vi "processMenuSelection.vi"(8 "eventData":T1, 10 "ItemPath":string, 11 "queues":T2) -> (0 "eventData 2":T1)   [LabVIEW 2018]
uses:
  Queues.ctl
  event data.ctl
  <vilib>/LabVIEW Targets/FPGA/cRIO/shared/nicrio_ModuleControls/nicrio_cRIO-9237_DataRatesRing.ctl
  supporting VIs/polymorphic VIs/enqueue for message handler.vi
  supporting VIs/polymorphic VIs/enqueue for user interface.vi
  supporting VIs/polymorphic VIs/enqueue for data processor.vi
  supporting VIs/polymorphic VIs/enqueue for file IO.vi
  RT/Message Handler loop/FPGA commands/RT - FPGA commands.lvlib
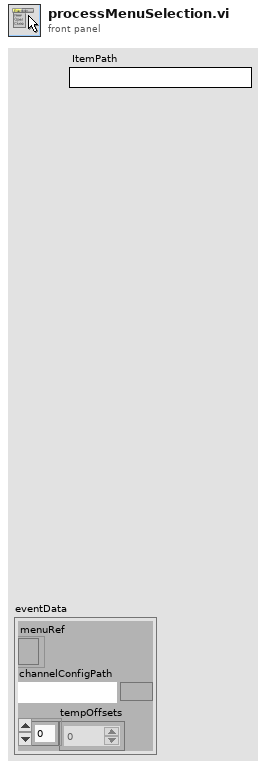
[diagram p1: front panel]
types:
  T1 = typedef "event data.ctl" = cluster{"menuRef":refnum<k9>, "channelConfigPath":path, "tempOffsets":dbl[]}
  T2 = typedef "Queues.ctl" = cluster{"messageHandler":refnum<queue>, "comms":refnum<queue>, "dataStream":refnum<queue>, "dataProcessor":refnum<queue>, "fileIO":refnum<queue>, "userInterface":refnum<queue>, "errors":refnum<queue>, "customCompressor":refnum<queue>}
  T3 = typedef "nicrio_cRIO-9237_DataRatesRing.ctl" = u8
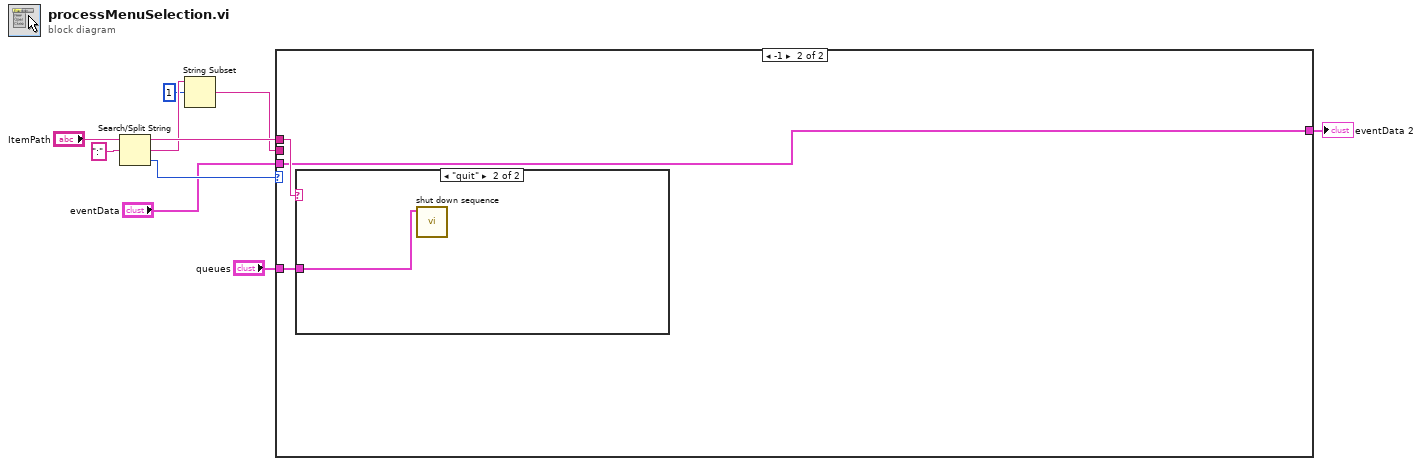
[diagram p0: block diagram]
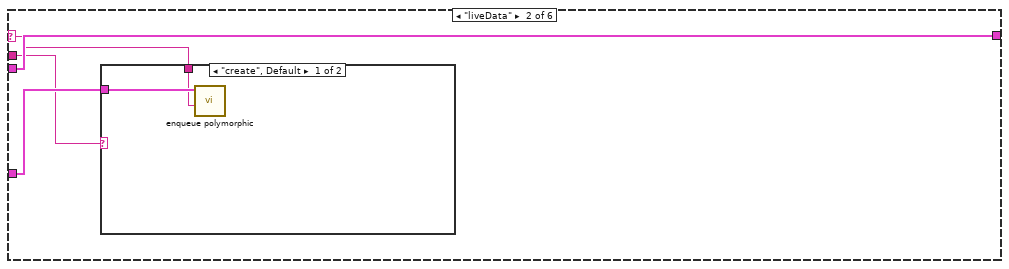
[diagram p3: hidden frame]
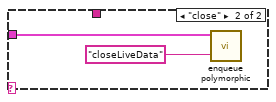
[diagram p4: hidden frame]
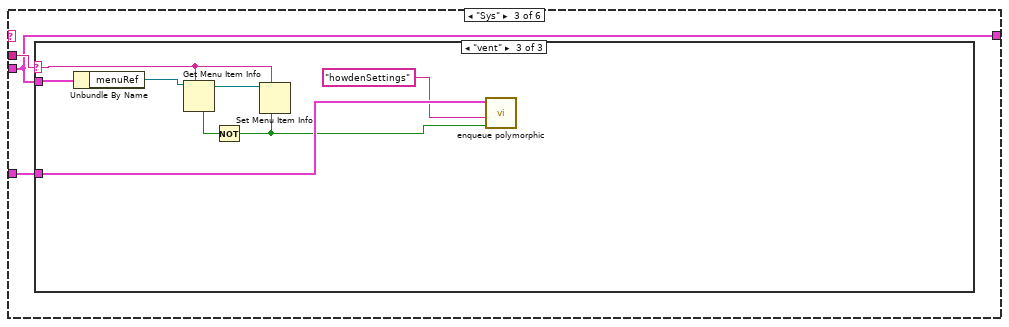
[diagram p5: hidden frame]
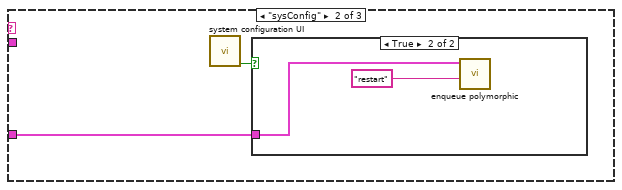
[diagram p7: hidden frame]
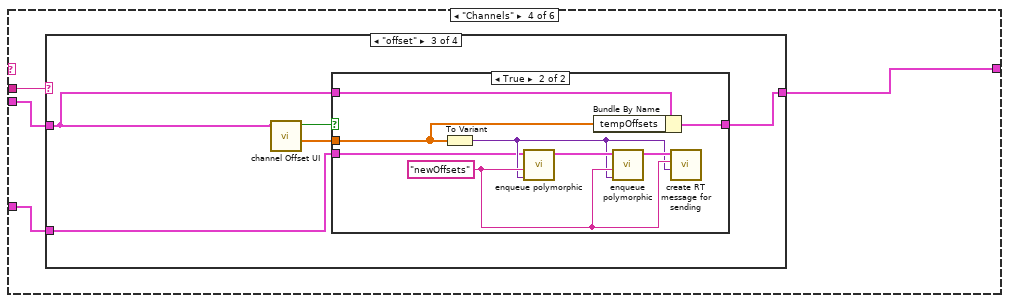
[diagram p9: hidden frame]
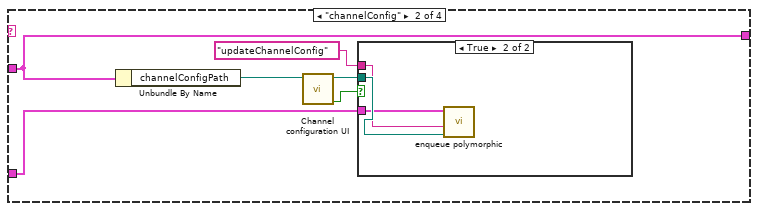
[diagram p11: hidden frame]
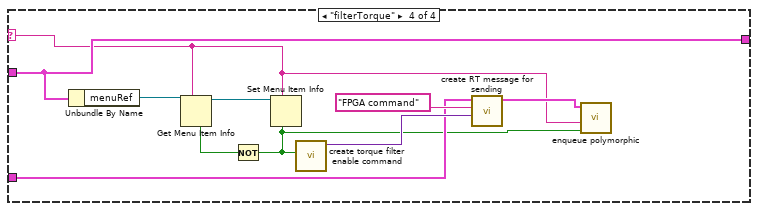
[diagram p14: hidden frame]
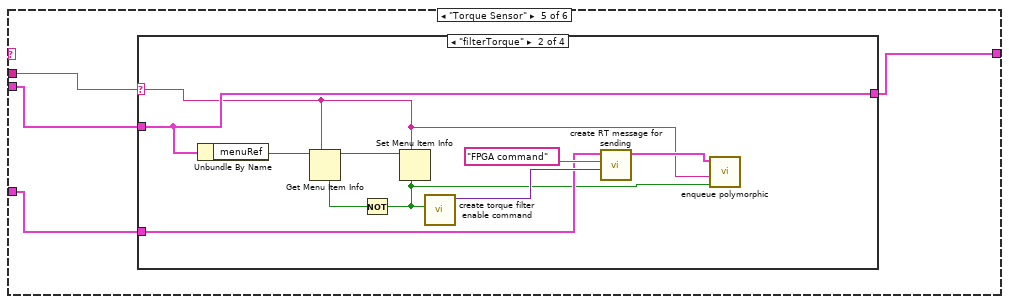
[diagram p15: hidden frame]
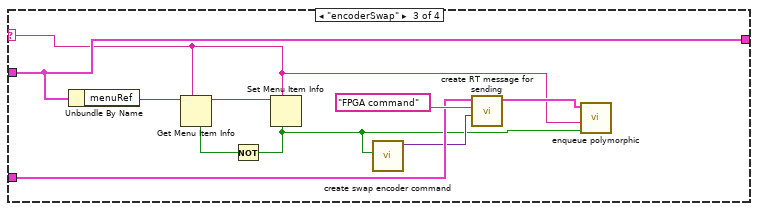
[diagram p17: hidden frame]
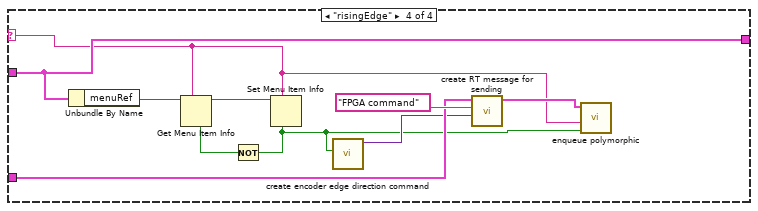
[diagram p18: hidden frame]
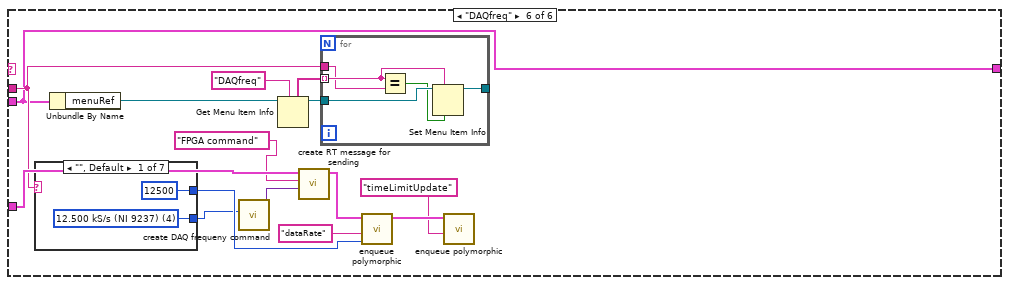
[diagram p19: hidden frame]
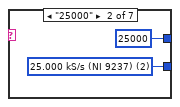
[diagram p20: hidden frame]
diagram:
  n1 = Search/Split String(string="ItemPath", search string/char (-)=":") -> (substring before match=w6:string, match + rest of string=w5:string, offset of match=w7:i32)  [unwired: 1 in]
  n2 = String Subset(string=w5, offset (0)=1) -> (substring=w3:string)  [unwired: 1 in]
  n3 = case shown="-1" w7 {
    tunnel: "queues" -> [w13 w149]
    tunnel: "eventData" -> [w12 w147]
    tunnel: w6 -> [w15 w148]
    tunnel: w3 -> [w14 _]
    tunnel: [w11 w147] -> w1
    frame 0, Default {
      n4 = case shown="\"\", Default" w15 {
        selector: w15 -> [_ w18 _ _ _ _]
        tunnel: w14 -> [_ w17 w26 w42 w79 w122]
        tunnel: w13 -> [_ w19 w27 w43 w81 w127]
        tunnel: w12 -> [w16 w20 w25 w41 w80 w121]
        tunnel: [w16 w20 w25 w40 w78 w121] -> w11
        frame "", Default {
        }
        frame "liveData" {
          n5 = case shown="\"create\", Default" w17 {
            tunnel: w19 -> [w22 w24]
            tunnel: w18 -> [w21 _]
            frame "create", Default {
              n6 = call-poly "enqueue polymorphic.vi"("message"=w21, "Queues"=w22) -> ()  [unwired: 9 in, 1 out]
            }
            frame "close" {
              n7 = call-poly "enqueue polymorphic.vi"("message"="closeLiveData", "Queues"=w24) -> ()  [unwired: 9 in, 1 out]
            }
          }
        }
        frame "Sys" {
          n8 = case shown="\"vent\"" w26 {
            selector: w26 -> [_ _ w34]
            tunnel: w27 -> [_ w28 w39]
            tunnel: w25 -> [_ _ w38]
            frame "", Default {
            }
            frame "sysConfig" {
              n9 = call "system configuration UI.vi"() -> ("file updated"=w29:bool)  [unwired: 11 in]
              n10 = case shown="True" w29 {
                tunnel: w28 -> [_ w30]
                frame False {
                }
                frame True {
                  n11 = call-poly "enqueue polymorphic.vi"("message"="restart" ("F button name (\"Cancel\")"), "Queues"=w30) -> ()  [unwired: 9 in, 1 out]
                }
              }
            }
            frame "vent" {
              n12 = Unbundle By Name(w38) -> ("menuRef"=w37:refnum<k9>)
              n13 = Get Menu Item Info(7:w34, 11:w37) -> (3:w32:refnum<k9>, 4:w35:bool)  [unwired: 1 in, 5 out]
              n14 = Not(x=w35) -> (.not. x?=w33:bool)
              n15 = Set Menu Item Info(6:w33, 7:w34, 11:w32) -> ()  [unwired: 4 in, 2 out]
              n16 = call-poly "enqueue polymorphic.vi"("data"=w33, "message"="howdenSettings" ("F button name (\"Cancel\")"), "Queues"=w39) -> ()  [unwired: 8 in, 1 out]
            }
          }
        }
        frame "Channels" {
          n17 = case shown="\"offset\"" w42 {
            selector: w42 -> [_ _ _ w70]
            tunnel: w43 -> [_ w46 w57 w72]
            tunnel: w41 -> [w44 w45 w54 w77]
            tunnel: [w44 w45 w55 w77] -> w40
            frame "", Default {
            }
            frame "channelConfig" {
              n18 = Unbundle By Name(w45) -> ("channelConfigPath"=w47:path)
              n19 = call "Channel configuration UI.vi"("config file"=w47) -> ("updated?"=w48:bool, "Current config file:"=w50:path)  [unwired: 9 in]
              n20 = case shown="True" w48 {
                tunnel: w50 -> [_ w53]
                tunnel: w46 -> [_ w52]
                tunnel: "updateChannelConfig" ("message") -> [_ w51]
                frame False {
                }
                frame True {
                  n21 = call-poly "enqueue polymorphic.vi"("data"=w53, "message"=w51, "Queues"=w52) -> ()  [unwired: 8 in, 1 out]
                }
              }
            }
            frame "offset" {
              n22 = call "channel Offset UI.vi"("eventData"=w54) -> ("offsets"=w56:dbl[], "changed?"=w58:bool)  [unwired: 9 in]
              n23 = case shown="True" w58 {
                tunnel: w56 -> [_ w60]
                tunnel: w57 -> [_ w63]
                tunnel: w54 -> [w59 w62]
                tunnel: [w59 w61] -> w55
                frame False {
                }
                frame True {
                  w65 = "newOffsets" ("message")
                  n24 = To Variant(anything=w60) -> (Variant=w64:variant)
                  n25 = call-poly "enqueue polymorphic.vi"("data"=w64, "message"=w65, "Queues"=w63) -> ("Queues out"=w67:T2)  [unwired: 8 in]
                  n26 = Bundle By Name(cluster=w62, "tempOffsets"=w60) -> (w61:T1)
                  n27 = call-poly "enqueue polymorphic.vi"("data"=w64, "message"=w65, "Queues"=w67) -> ("Queues out"=w66:T2)  [unwired: 8 in]
                  n28 = call "create RT message for sending.vi"("RT data"=w64, "RT message"=w65, "Queues in"=w66) -> ()  [unwired: 8 in, 1 out]
                }
              }
            }
            frame "filterTorque" {
              n29 = Unbundle By Name(w77) -> ("menuRef"=w68:refnum<k9>)
              n30 = Get Menu Item Info(7:w70, 11:w68) -> (3:w75:refnum<k9>, 4:w76:bool)  [unwired: 1 in, 5 out]
              n31 = Not(x=w76) -> (.not. x?=w69:bool)
              n32 = Set Menu Item Info(6:w69, 7:w70, 11:w75) -> ()  [unwired: 4 in, 2 out]
              n33 = call "create torque filter enable command.vi"("Enable filter"=w69) -> ("command message"=w74:variant)  [unwired: 10 in]
              n34 = call "create RT message for sending.vi"("RT data"=w74, "RT message"="FPGA command", "Queues in"=w72) -> ("Queues out"=w71:T2)  [unwired: 8 in]
              n35 = call-poly "enqueue polymorphic.vi"("data"=w69, "message"=w70, "Queues"=w71) -> ()  [unwired: 8 in, 1 out]
            }
          }
        }
        frame "Torque Sensor" {
          n36 = case shown="\"filterTorque\"" w79 {
            selector: w79 -> [_ w84 w95 w105]
            tunnel: w81 -> [_ w86 w97 w107]
            tunnel: w80 -> [w82 w92 w102 w112]
            tunnel: [w82 w92 w102 w112] -> w78
            frame "", Default {
            }
            frame "filterTorque" {
              n37 = Unbundle By Name(w92) -> ("menuRef"=w91:refnum<k9>)
              n38 = Get Menu Item Info(7:w84, 11:w91) -> (3:w89:refnum<k9>, 4:w90:bool)  [unwired: 1 in, 5 out]
              n39 = Not(x=w90) -> (.not. x?=w83:bool)
              n40 = Set Menu Item Info(6:w83, 7:w84, 11:w89) -> ()  [unwired: 4 in, 2 out]
              n41 = call "create torque filter enable command.vi"("Enable filter"=w83) -> ("command message"=w88:variant)  [unwired: 10 in]
              n42 = call "create RT message for sending.vi"("RT data"=w88, "RT message"="FPGA command", "Queues in"=w86) -> ("Queues out"=w85:T2)  [unwired: 8 in]
              n43 = call-poly "enqueue polymorphic.vi"("data"=w83, "message"=w84, "Queues"=w85) -> ()  [unwired: 8 in, 1 out]
            }
            frame "encoderSwap" {
              n44 = Unbundle By Name(w102) -> ("menuRef"=w101:refnum<k9>)
              n45 = Get Menu Item Info(7:w95, 11:w101) -> (3:w99:refnum<k9>, 4:w100:bool)  [unwired: 1 in, 5 out]
              n46 = Not(x=w100) -> (.not. x?=w93:bool)
              n47 = Set Menu Item Info(6:w93, 7:w95, 11:w99) -> ()  [unwired: 4 in, 2 out]
              n48 = call "create swap encoder command.vi"("swap encoders"=w93) -> ("command message"=w94:variant)  [unwired: 10 in]
              n49 = call "create RT message for sending.vi"("RT data"=w94, "RT message"="FPGA command", "Queues in"=w97) -> ("Queues out"=w96:T2)  [unwired: 8 in]
              n50 = call-poly "enqueue polymorphic.vi"("data"=w93, "message"=w95, "Queues"=w96) -> ()  [unwired: 8 in, 1 out]
            }
            frame "risingEdge" {
              n51 = Unbundle By Name(w112) -> ("menuRef"=w111:refnum<k9>)
              n52 = Get Menu Item Info(7:w105, 11:w111) -> (3:w109:refnum<k9>, 4:w110:bool)  [unwired: 1 in, 5 out]
              n53 = Not(x=w110) -> (.not. x?=w103:bool)
              n54 = Set Menu Item Info(6:w103, 7:w105, 11:w109) -> ()  [unwired: 4 in, 2 out]
              n55 = call "create encoder edge direction command.vi"("Falling edge?"=w103) -> ("command message"=w104:variant)  [unwired: 10 in]
              n56 = call "create RT message for sending.vi"("RT data"=w104, "RT message"="FPGA command", "Queues in"=w107) -> ("Queues out"=w106:T2)  [unwired: 8 in]
              n57 = call-poly "enqueue polymorphic.vi"("data"=w103, "message"=w105, "Queues"=w106) -> ()  [unwired: 8 in, 1 out]
            }
          }
        }
        frame "DAQfreq" {
          n58 = case shown="\"\", Default" w122 {
            tunnel: [u16 12500 u16 25000 u16 12500 u16 10000 u16 5000 u16 2500 u16 2000] -> w120
            tunnel: [w134 w135 w137 w140 w141 w143 w145] -> w117
            frame "", Default {
              w134 = T3 4 items=["50.000 kS/s (NI 9237)"=1, "25.000 kS/s (NI 9237)"=2, "16.667 kS/s (NI 9237)"=3, "12.500 kS/s (NI 9237)"=4, "10.000 kS/s (NI 9237)"=5, "8.333 kS/s (NI 9237)"=6, "7.143 kS/s (NI 9237)"=7, "6.250 kS/s (NI 9237)"=8, "5.556 kS/s (NI 9237)"=9, "5.000 kS/s (NI 9237)"=10, "4.545 kS/s (NI 9237)"=11, "4.167 kS/s (NI 9237)"=12, "3.846 kS/s (NI 9237)"=13, "3.571 kS/s (NI 9237)"=14, "3.333 kS/s (NI 9237)"=15, "3.125 kS/s (NI 9237)"=16, "2.941 kS/s (NI 9237)"=17, "2.778 kS/s (NI 9237)"=18, "2.632 kS/s (NI 9237)"=19, "2.500 kS/s (NI 9237)"=20, "2.381 kS/s (NI 9237)"=21, "2.273 kS/s (NI 9237)"=22, "2.174 kS/s (NI 9237)"=23, "2.083 kS/s (NI 9237)"=24, "2.000 kS/s (NI 9237)"=25, "1.923 kS/s (NI 9237)"=26, "1.852 kS/s (NI 9237)"=27, "1.786 kS/s (NI 9237)"=28, "1.724 kS/s (NI 9237)"=29, "1.667 kS/s (NI 9237)"=30, "1.613 kS/s (NI 9237)"=31] ("Data Rate")
            }
            frame "25000" {
              w135 = T3 2 items=["50.000 kS/s (NI 9237)"=1, "25.000 kS/s (NI 9237)"=2, "16.667 kS/s (NI 9237)"=3, "12.500 kS/s (NI 9237)"=4, "10.000 kS/s (NI 9237)"=5, "8.333 kS/s (NI 9237)"=6, "7.143 kS/s (NI 9237)"=7, "6.250 kS/s (NI 9237)"=8, "5.556 kS/s (NI 9237)"=9, "5.000 kS/s (NI 9237)"=10, "4.545 kS/s (NI 9237)"=11, "4.167 kS/s (NI 9237)"=12, "3.846 kS/s (NI 9237)"=13, "3.571 kS/s (NI 9237)"=14, "3.333 kS/s (NI 9237)"=15, "3.125 kS/s (NI 9237)"=16, "2.941 kS/s (NI 9237)"=17, "2.778 kS/s (NI 9237)"=18, "2.632 kS/s (NI 9237)"=19, "2.500 kS/s (NI 9237)"=20, "2.381 kS/s (NI 9237)"=21, "2.273 kS/s (NI 9237)"=22, "2.174 kS/s (NI 9237)"=23, "2.083 kS/s (NI 9237)"=24, "2.000 kS/s (NI 9237)"=25, "1.923 kS/s (NI 9237)"=26, "1.852 kS/s (NI 9237)"=27, "1.786 kS/s (NI 9237)"=28, "1.724 kS/s (NI 9237)"=29, "1.667 kS/s (NI 9237)"=30, "1.613 kS/s (NI 9237)"=31] ("Data Rate")
            }
            frame "12500" {
              w137 = T3 4 items=["50.000 kS/s (NI 9237)"=1, "25.000 kS/s (NI 9237)"=2, "16.667 kS/s (NI 9237)"=3, "12.500 kS/s (NI 9237)"=4, "10.000 kS/s (NI 9237)"=5, "8.333 kS/s (NI 9237)"=6, "7.143 kS/s (NI 9237)"=7, "6.250 kS/s (NI 9237)"=8, "5.556 kS/s (NI 9237)"=9, "5.000 kS/s (NI 9237)"=10, "4.545 kS/s (NI 9237)"=11, "4.167 kS/s (NI 9237)"=12, "3.846 kS/s (NI 9237)"=13, "3.571 kS/s (NI 9237)"=14, "3.333 kS/s (NI 9237)"=15, "3.125 kS/s (NI 9237)"=16, "2.941 kS/s (NI 9237)"=17, "2.778 kS/s (NI 9237)"=18, "2.632 kS/s (NI 9237)"=19, "2.500 kS/s (NI 9237)"=20, "2.381 kS/s (NI 9237)"=21, "2.273 kS/s (NI 9237)"=22, "2.174 kS/s (NI 9237)"=23, "2.083 kS/s (NI 9237)"=24, "2.000 kS/s (NI 9237)"=25, "1.923 kS/s (NI 9237)"=26, "1.852 kS/s (NI 9237)"=27, "1.786 kS/s (NI 9237)"=28, "1.724 kS/s (NI 9237)"=29, "1.667 kS/s (NI 9237)"=30, "1.613 kS/s (NI 9237)"=31] ("Data Rate")
            }
            frame "10000" {
              w140 = T3 5 items=["50.000 kS/s (NI 9237)"=1, "25.000 kS/s (NI 9237)"=2, "16.667 kS/s (NI 9237)"=3, "12.500 kS/s (NI 9237)"=4, "10.000 kS/s (NI 9237)"=5, "8.333 kS/s (NI 9237)"=6, "7.143 kS/s (NI 9237)"=7, "6.250 kS/s (NI 9237)"=8, "5.556 kS/s (NI 9237)"=9, "5.000 kS/s (NI 9237)"=10, "4.545 kS/s (NI 9237)"=11, "4.167 kS/s (NI 9237)"=12, "3.846 kS/s (NI 9237)"=13, "3.571 kS/s (NI 9237)"=14, "3.333 kS/s (NI 9237)"=15, "3.125 kS/s (NI 9237)"=16, "2.941 kS/s (NI 9237)"=17, "2.778 kS/s (NI 9237)"=18, "2.632 kS/s (NI 9237)"=19, "2.500 kS/s (NI 9237)"=20, "2.381 kS/s (NI 9237)"=21, "2.273 kS/s (NI 9237)"=22, "2.174 kS/s (NI 9237)"=23, "2.083 kS/s (NI 9237)"=24, "2.000 kS/s (NI 9237)"=25, "1.923 kS/s (NI 9237)"=26, "1.852 kS/s (NI 9237)"=27, "1.786 kS/s (NI 9237)"=28, "1.724 kS/s (NI 9237)"=29, "1.667 kS/s (NI 9237)"=30, "1.613 kS/s (NI 9237)"=31] ("Data Rate")
            }
            frame "5000" {
              w141 = T3 10 items=["50.000 kS/s (NI 9237)"=1, "25.000 kS/s (NI 9237)"=2, "16.667 kS/s (NI 9237)"=3, "12.500 kS/s (NI 9237)"=4, "10.000 kS/s (NI 9237)"=5, "8.333 kS/s (NI 9237)"=6, "7.143 kS/s (NI 9237)"=7, "6.250 kS/s (NI 9237)"=8, "5.556 kS/s (NI 9237)"=9, "5.000 kS/s (NI 9237)"=10, "4.545 kS/s (NI 9237)"=11, "4.167 kS/s (NI 9237)"=12, "3.846 kS/s (NI 9237)"=13, "3.571 kS/s (NI 9237)"=14, "3.333 kS/s (NI 9237)"=15, "3.125 kS/s (NI 9237)"=16, "2.941 kS/s (NI 9237)"=17, "2.778 kS/s (NI 9237)"=18, "2.632 kS/s (NI 9237)"=19, "2.500 kS/s (NI 9237)"=20, "2.381 kS/s (NI 9237)"=21, "2.273 kS/s (NI 9237)"=22, "2.174 kS/s (NI 9237)"=23, "2.083 kS/s (NI 9237)"=24, "2.000 kS/s (NI 9237)"=25, "1.923 kS/s (NI 9237)"=26, "1.852 kS/s (NI 9237)"=27, "1.786 kS/s (NI 9237)"=28, "1.724 kS/s (NI 9237)"=29, "1.667 kS/s (NI 9237)"=30, "1.613 kS/s (NI 9237)"=31] ("Data Rate")
            }
            frame "2500" {
              w143 = T3 20 items=["50.000 kS/s (NI 9237)"=1, "25.000 kS/s (NI 9237)"=2, "16.667 kS/s (NI 9237)"=3, "12.500 kS/s (NI 9237)"=4, "10.000 kS/s (NI 9237)"=5, "8.333 kS/s (NI 9237)"=6, "7.143 kS/s (NI 9237)"=7, "6.250 kS/s (NI 9237)"=8, "5.556 kS/s (NI 9237)"=9, "5.000 kS/s (NI 9237)"=10, "4.545 kS/s (NI 9237)"=11, "4.167 kS/s (NI 9237)"=12, "3.846 kS/s (NI 9237)"=13, "3.571 kS/s (NI 9237)"=14, "3.333 kS/s (NI 9237)"=15, "3.125 kS/s (NI 9237)"=16, "2.941 kS/s (NI 9237)"=17, "2.778 kS/s (NI 9237)"=18, "2.632 kS/s (NI 9237)"=19, "2.500 kS/s (NI 9237)"=20, "2.381 kS/s (NI 9237)"=21, "2.273 kS/s (NI 9237)"=22, "2.174 kS/s (NI 9237)"=23, "2.083 kS/s (NI 9237)"=24, "2.000 kS/s (NI 9237)"=25, "1.923 kS/s (NI 9237)"=26, "1.852 kS/s (NI 9237)"=27, "1.786 kS/s (NI 9237)"=28, "1.724 kS/s (NI 9237)"=29, "1.667 kS/s (NI 9237)"=30, "1.613 kS/s (NI 9237)"=31] ("Data Rate")
            }
            frame "2000" {
              w145 = T3 25 items=["50.000 kS/s (NI 9237)"=1, "25.000 kS/s (NI 9237)"=2, "16.667 kS/s (NI 9237)"=3, "12.500 kS/s (NI 9237)"=4, "10.000 kS/s (NI 9237)"=5, "8.333 kS/s (NI 9237)"=6, "7.143 kS/s (NI 9237)"=7, "6.250 kS/s (NI 9237)"=8, "5.556 kS/s (NI 9237)"=9, "5.000 kS/s (NI 9237)"=10, "4.545 kS/s (NI 9237)"=11, "4.167 kS/s (NI 9237)"=12, "3.846 kS/s (NI 9237)"=13, "3.571 kS/s (NI 9237)"=14, "3.333 kS/s (NI 9237)"=15, "3.125 kS/s (NI 9237)"=16, "2.941 kS/s (NI 9237)"=17, "2.778 kS/s (NI 9237)"=18, "2.632 kS/s (NI 9237)"=19, "2.500 kS/s (NI 9237)"=20, "2.381 kS/s (NI 9237)"=21, "2.273 kS/s (NI 9237)"=22, "2.174 kS/s (NI 9237)"=23, "2.083 kS/s (NI 9237)"=24, "2.000 kS/s (NI 9237)"=25, "1.923 kS/s (NI 9237)"=26, "1.852 kS/s (NI 9237)"=27, "1.786 kS/s (NI 9237)"=28, "1.724 kS/s (NI 9237)"=29, "1.667 kS/s (NI 9237)"=30, "1.613 kS/s (NI 9237)"=31] ("Data Rate")
            }
          }
          n59 = Unbundle By Name(w121) -> ("menuRef"=w123:refnum<k9>)
          n60 = call "create DAQ frequeny command.vi"("Data Rate"=w117) -> ("command message"=w116:variant)  [unwired: 10 in]
          n61 = Get Menu Item Info(7:"DAQfreq" ("item tag"), 11:w123) -> (3:w124:refnum<k9>, 5:w125:string[])  [unwired: 1 in, 5 out]
          n62 = call "create RT message for sending.vi"("RT data"=w116, "RT message"="FPGA command", "Queues in"=w127) -> ("Queues out"=w119:T2)  [unwired: 8 in]
          n63 = for {
            tunnel: w125 -> [w130] mode=indexing
            tunnel: w124 -> [w132]
            tunnel: [w131] -> _
            tunnel: w122 -> [w128]
            n64 = Equal?(x=w130, y=w128) -> (x = y?=w129:bool)
            n65 = Set Menu Item Info(6:w129, 7:w130, 11:w132) -> (3:w131:refnum<k9>)  [unwired: 4 in, 1 out]
          }
          n66 = call-poly "enqueue polymorphic.vi"("data"=w120, "message"="dataRate", "Queues"=w119) -> ("Queues out"=w114:T2)  [unwired: 8 in]
          n67 = call-poly "enqueue polymorphic.vi"("message"="timeLimitUpdate", "Queues"=w114) -> ()  [unwired: 9 in, 1 out]
        }
      }
    }
    frame -1 {
      n68 = case shown="\"quit\"" w148 {
        tunnel: w149 -> [_ w150]
        frame "False", Default {
        }
        frame "quit" {
          n69 = call "shut down sequence.vi"("queues"=w150) -> ()  [unwired: 11 in]
        }
      }
    }
  }
  "eventData 2" <- w1
